vi "getHeater.vi"(6 "Channel":i32, 8 "error in (no error)":errorcluster, 11 "Instrument.Cryostat in":refnum<class "Instrument.Cryostat.lvclass">) -> (0 "error out":errorcluster, 1 "Status":string, 2 "Current (A)":dbl, 3 "Instrument.Cryostat out":refnum<class "Instrument.Cryostat.lvclass">)   [LabVIEW 2019, in "Instrument.Cryostat.lvclass"]
uses:
  Instrument.Cryostat.lvclass
  Typedefs/getHeater--cluster.ctl
  Typedefs/Cryostat.commands--enum.ctl
  69337c34-fda4-4886-b877-cdf307779210.vi
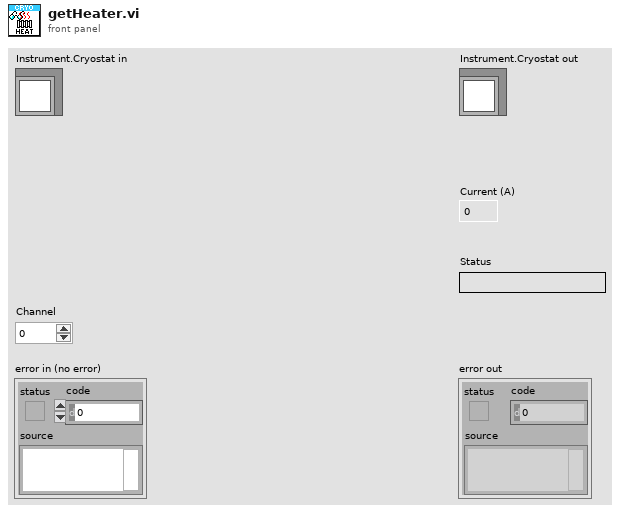
[diagram p1: front panel]
types:
  T1 = typedef "Instrument.Cryostat.lvclass/Cryostat.commands--enum.ctl" = enum16{"getLN2Level", "getLHeLevel", "getMagnet", "getMagnetVector", "setMagnet", "setMagnetVector", "getAngle", "setAngle", "getTemperature", "setTemperature", "getHeater", "setHeater", "getChamber", "setChamber", "getPressure"}
  T2 = typedef "Instrument.Cryostat.lvclass/getHeater--cluster.ctl" = cluster{"current":dbl, "status":string}
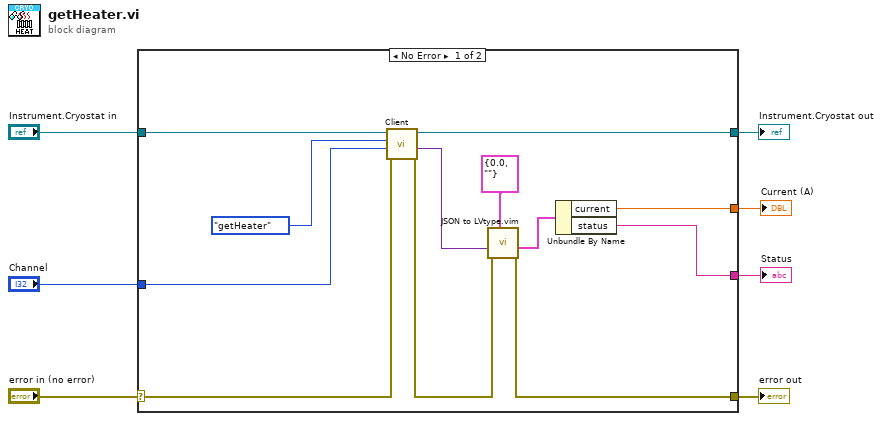
[diagram p0: block diagram]
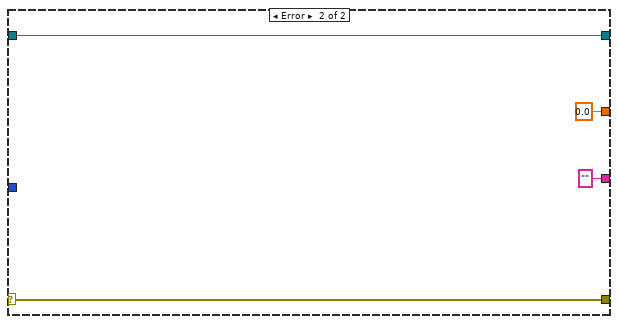
[diagram p2: hidden frame]
diagram:
  n1 = case shown="No Error" "error in (no error)" {
    selector: "error in (no error)" -> [w14 w23]
    tunnel: [w8 w23] -> w6
    tunnel: [w19 w22] -> w4
    tunnel: "Instrument.Cryostat in" -> [w13 w22]
    tunnel: [w18 0.0 ("Current")] -> w3
    tunnel: [w17 "" ("Status")] -> w2
    tunnel: "Channel" -> [w16 _]
    frame No Error {
      n2 = call-dynamic "Client.vi"("error in (no error)"=w14, "Data in"=w16, "Command in"=Cryostat.commands--enum."getHeater" ("commands"), "Instrument in"=w13) -> ("error out"=w9:errorcluster, "Data out"=w11:variant, "Instrument out"=w19:refnum<class "Instrument.Cryostat.lvclass">)  [unwired: 4 in, 1 out]
      n3 = call "JSON to LVtype.vim"("type"=T2 {"current"=0.0, "status"=""} ("getHeat"), "error in (no error)"=w9, "JSON Data in"=w11) -> ("error out"=w8:errorcluster, "Data out"=w10:T2)  [unwired: 7 in]
      n4 = Unbundle By Name(w10) -> ("current"=w18:dbl, "status"=w17:string)
    }
    frame Error {
    }
  }
  "error out" <- w6
  "Instrument.Cryostat out" <- w4
  "Current (A)" <- w3
  "Status" <- w2
